vi "_UpdateListSelection.vi"(7 "Refs":T2, 9 "Action in":T1 caption="Action", 10 "Display State In in":T3 caption="State", 11 "Data In in":T6) -> (1 "Action out":T1 caption="Action", 2 "Display State In out":T3 caption="State", 3 "Data In out":T6)   [LabVIEW 2013, in "UI_TimeSelector.xctl"]
uses:
  UI_TimeSelector.xctl
  Data.ctl
  State.ctl
  Typedefs/INTERNAL-DATA.ctl
  Interface/DEF-Mode.ctl
  Typedefs/INTERNAL-REFs.ctl
  <vilib>/_xctls/Action.ctl
  <vilib>/_xctls/XControlSupport.lvlib
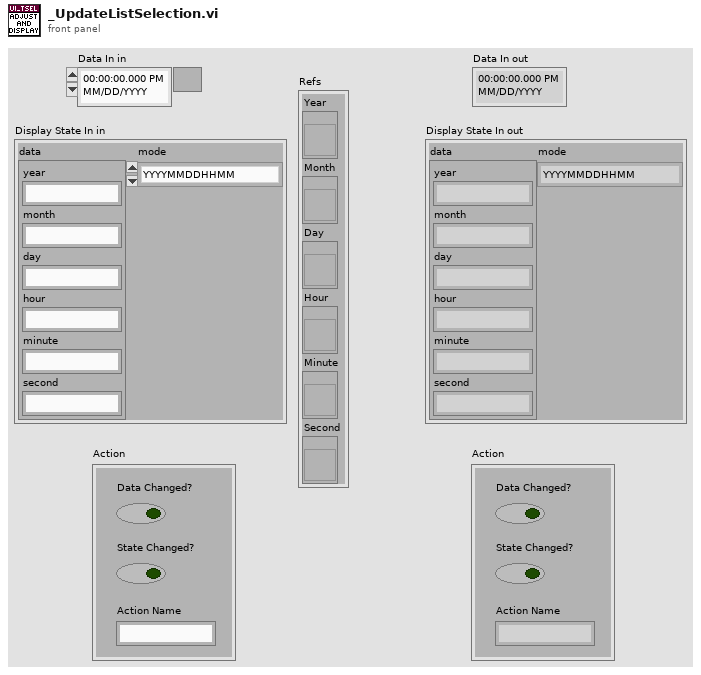
[diagram p1: front panel]
types:
  T1 = typedef "XControlSupport.lvlib/Action.ctl" = cluster{"Data Changed?":bool, "State Changed?":bool, "Action Name":string}
  T2 = typedef "UI_TimeSelector.xctl/INTERNAL-REFs.ctl" = cluster{"Year":refnum<vi>, "Month":refnum<vi>, "Day":refnum<vi>, "Hour":refnum<vi>, "Minute":refnum<vi>, "Second":refnum<vi>}
  T3 = typedef "UI_TimeSelector.xctl/State.ctl" = cluster{"data":T4, "mode":T5}
  T4 = typedef "UI_TimeSelector.xctl/INTERNAL-DATA.ctl" = cluster{"year":string, "month":string, "day":string, "hour":string, "minute":string, "second":string}
  T5 = typedef "UI_TimeSelector.xctl/DEF-Mode.ctl" = enum16{"YYYYMMDDHHMM", "YYYYMMDDHHMMSS", "YYYY", "YYYYMM", "YYYYMMDD", "HHMM", "HHMMSS"}
  T6 = typedef "UI_TimeSelector.xctl/Data.ctl" = timestamp
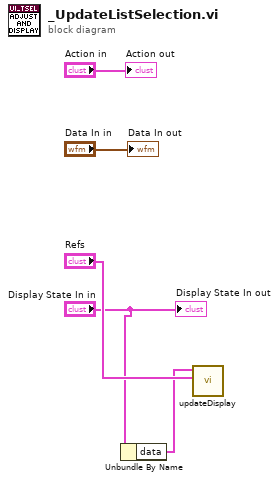
[diagram p0: block diagram]
diagram:
  n1 = Unbundle By Name("Display State In in") -> ("data"=w1:T4)
  n2 = call "updateDisplay.vi"("display refs"="Refs", "data"=w1) -> ()  [unwired: 9 in, 1 out]
  "Data In out" <- "Data In in"
  "Display State In out" <- "Display State In in"
  "Action out" <- "Action in"
